vi "cover_CSVBackslash.vi"(11 "String in":string) -> (3 "String out":string)   [LabVIEW 2017]
panel:
  # "This for Step vi"
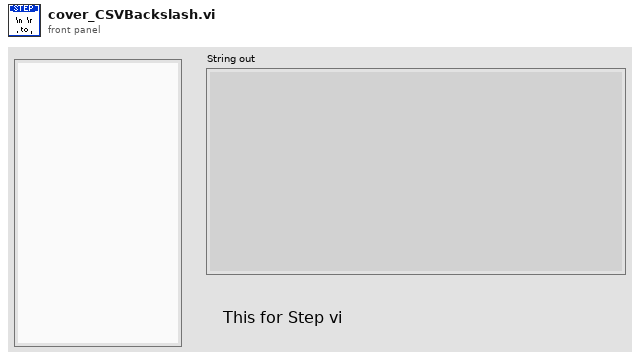
[diagram p1: front panel]
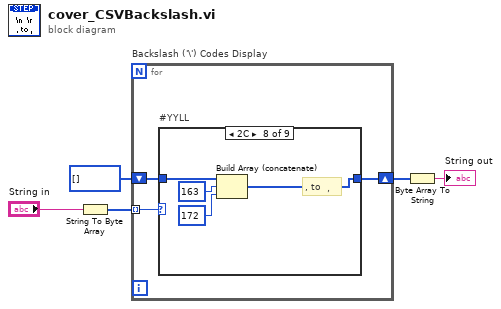
[diagram p0: block diagram]
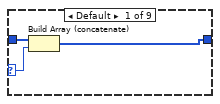
[diagram p2: hidden frame]
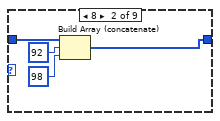
[diagram p3: hidden frame]
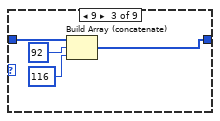
[diagram p4: hidden frame]
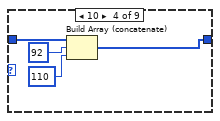
[diagram p5: hidden frame]
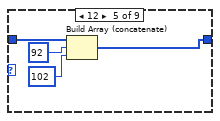
[diagram p6: hidden frame]
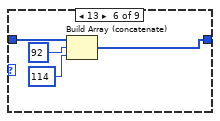
[diagram p7: hidden frame]
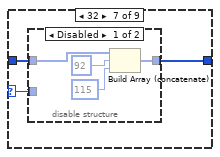
[diagram p8: hidden frame]
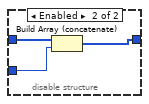
[diagram p9: hidden frame]
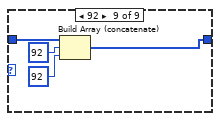
[diagram p10: hidden frame]
diagram:
  n1 = String To Byte Array(string="String in") -> (unsigned byte array=w3:u8[])
  n2 = for "Backslash ('\\') Codes Display" {
    tunnel: w3 -> [w8] mode=indexing
    shift-right: [w7] -> w2
    shift-left: u8[] [] ("unsigned byte array") -> [w6]
    n3 = case "#YYLL" shown="2C" w8 {
      selector: w8 -> [w9 _ _ _ _ _ w32 _ _]
      tunnel: [w10 w14 w18 w22 w26 w30 w33 w44 w48] -> w7
      tunnel: w6 -> [w11 w15 w19 w23 w27 w31 w34 w45 w49]
      frame Default {
        n4 = Build Array (concatenate)(w11, w9) -> (w10:u8[])
      }
      frame 8 {
        n5 = Build Array (concatenate)(w15, u8 92, u8 98) -> (w14:u8[])
      }
      frame 9 {
        n6 = Build Array (concatenate)(w19, u8 92, u8 116) -> (w18:u8[])
      }
      frame 10 {
        n7 = Build Array (concatenate)(w23, u8 92, u8 110) -> (w22:u8[])
      }
      frame 12 {
        n8 = Build Array (concatenate)(w27, u8 92, u8 102) -> (w26:u8[])
      }
      frame 13 {
        n9 = Build Array (concatenate)(w31, u8 92, u8 114) -> (w30:u8[])
      }
      frame 32 {
        n10 = disable-structure shown="Disabled" {
          disable-tunnel: w34 -> [w38 w41]
          disable-tunnel: [w37 w40] -> w33
          disable-tunnel: w32 -> [_ w39]
          frame Disabled {
            n11 = Build Array (concatenate)(w38, u8 92, u8 115) -> (w37:u8[])
          }
          frame Enabled {
            n12 = Build Array (concatenate)(w41, w39) -> (w40:u8[])
          }
        }
      }
      frame 44 {
        # ", to ，"
        n13 = Build Array (concatenate)(w45, u8 163, u8 172) -> (w44:u8[])
      }
      frame 92 {
        n14 = Build Array (concatenate)(w49, u8 92, u8 92) -> (w48:u8[])
      }
    }
  }
  n15 = Byte Array To String(unsigned byte array=w2) -> (string=→"String out":string)
